vi "FpgaLink_Check_Comm.vi"(8 "error in (no error)":errorcluster, 11 "handle":i64) -> (0 "error out":errorcluster, 2 "Is Capable?":bool, 3 "handle out":i64)   [LabVIEW 2011]
doc: "Check to see if the device supports CommFPGA.\n\nCommFPGA is a simple channel read/write protocol using USB bulk endpoints 6 and 8. This only returns whether the micro itself supports the protocol, not whether the target logic device has been configured with a suitable design implementing the other end of the protocol. An affirmative response means you are free to call flReadChannel(), flWriteChannel() and flIsFPGARunning()."
uses:
  libfpgalink.dll
panel:
  out "bool":u8
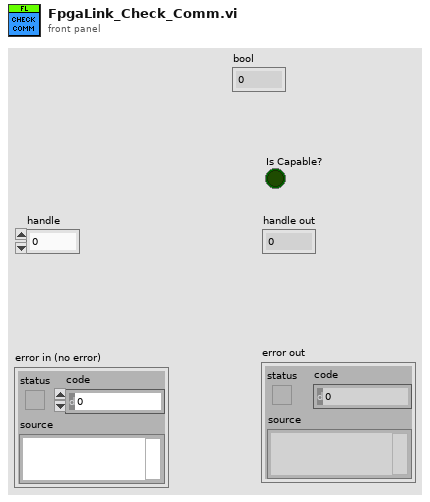
[diagram p1: front panel]
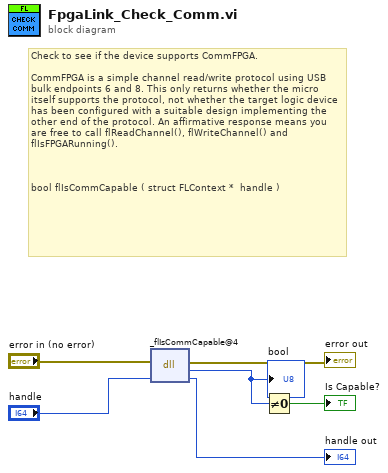
[diagram p0: block diagram]
diagram:
  # "Check to see if the device supports CommFPGA.\n\nCommFPGA is a simple channel read/write protocol using USB bulk endpoints 6 and 8. This only returns whether the micro itself supports the protocol, not whether the target logic device has been configured with a suitable design implementing the other end of the protocol. An affirmative response means you are free to call flReadChannel(), flWriteChannel() and flIsFPGARunning().\n\n\n\nbool flIsCommCapable\t(\tstruct FLContext * \thandle\t)"
  n1 = dll-call lib="libfpgalink.*" fn="_flIsCommCapable@4"(error in="error in (no error)", "handle"="handle") -> (error out=→"error out":errorcluster, "bool"=w3:u8, "handle"=→"handle out":i64)  [unwired: 2 in, 1 out]
  "bool" <- w3
  n2 = Not Equal To 0?(x=w3) -> (x != 0?=→"Is Capable?":bool)
